vi "LVClasse_Intensity ctor from Pupil.vi"(0 "Intensity (const)":refnum<class "Intensity.lvclass">, 5 "Pupil":refnum<class "Pupil.lvclass">, 7 "coef":sgl, 11 "error in (no error)":errorcluster) -> (4 "Intensity (new)":refnum<class "Intensity.lvclass">, 6 "Pupil (dup)":refnum<class "Pupil.lvclass">, 15 "error out":errorcluster)   [LabVIEW 2020, in "Intensity.lvclass"]
doc: "Phase constructor from pupil.\n\n--------------------------------------------------------------------------------\n\n<B>PhaseIn </B> : Constant Pointer to Phase object.\n<B>PhaseOut </B> : Constant Pointer to Phase object.\n<B>Pupil </B> : pupil object.\n<B>default_value </B> : Phase default value.\n<B>ErrorIn </B> : Error\n<B>ErrorOut </B> : Error\n\n--------------------------------------------------------------------------------"
uses:
  Intensity.lvclass
  Pupil/Pupil.lvclass
  Controls/Handle creation.ctl
  Intensity.lvclass/Intensity.ctl
  Pupil/LVClass_Pupil Read Pupil.vi
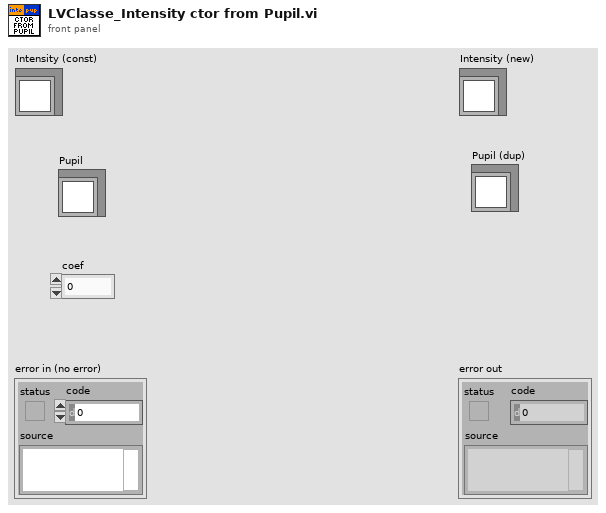
[diagram p1: front panel]
types:
  T1 = typedef "Handle creation.ctl" = enum16{"By ctor", "By write function"}
  T2 = typedef "ClassID.ctl" = i64
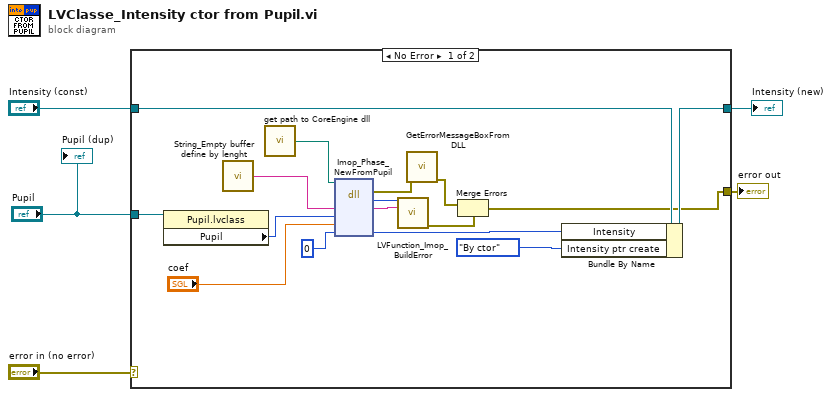
[diagram p0: block diagram]
diagram:
  n1 = case shown="No Error" "error in (no error)" {
    selector: "error in (no error)" -> [_ w23]
    tunnel: [w6 w23] -> w4
    tunnel: [w12 w22] -> w2
    tunnel: "Intensity (const)" -> [w13 w22]
    tunnel: "Pupil" -> [w11 _]
    frame No Error {
      n2 = property class="Pupil.lvclass"(reference=w11) -> ("Pupil"=w10:T2)  [unwired: 1 in, 2 out]
      n3 = call "String_Empty buffer define by lenght.vi"() -> ("Empty buffer"=w18:string)  [unwired: 1 in]
      n4 = call "get path to CoreEngine dll.vi"() -> ("path to wavekit library"=w17:path)  [unwired: 14 in, 1 out]
      n5 = dll-call lib="D:/soft/HASO_v3/SVN_trunk/ImOpCoreEngine4_LV2011/DLLs/c_interface_vc100.dll" fn="Imop_Phase_NewFromPupil"(path in=w17, "message"=w18, "pupil"=w10, "coef"="coef", "phase"=0 ("objet")) -> (error out=w16:errorcluster, "return type"=w21:i32, "message"=w20:string, "phase"=w19:i64)  [unwired: 4 in, 1 out]
      n6 = call "LVFunction_Imop_BuildError.vi"("code"=w21, "String to Prepend to source (\"\")"=w20) -> ("error out"=w7:errorcluster)  [unwired: 13 in]
      n7 = call "GetErrorMessageBoxFromDLL.vi"("error IN"=w16) -> ("error OUT"=w8:errorcluster)  [unwired: 10 in]
      n8 = Merge Errors(w8, w7) -> (w6:errorcluster)
      n9 = Bundle By Name(cluster=w13, "Intensity"=w19, "Intensity ptr create"=Handle_creation."By ctor" ("HasoData ptr create")) -> (w12:refnum<class "Intensity.lvclass">)
    }
    frame Error {
    }
  }
  "error out" <- w4
  "Intensity (new)" <- w2
  "Pupil (dup)" <- "Pupil"
